vi "Limit Testing Frequency.vi"(6 "limit test config":T2={"pass region"=0, "include UL"=TRUE, "include LL"=TRUE} {"pass region" items=["inside limits", "outside limits"]}, 8 "error in (no error)":errorcluster, 9 "lower limit":cluster{"x0":dbl, "dx":dbl, "Y":dbl[]}={"x0"=0.0, "dx"=1.0, "Y"=[]} {"Y" format="%.2p"; "dx" format="%.2p"; "x0" format="%.2p"}, 10 "upper limit":cluster{"x0":dbl, "dx":dbl, "Y":dbl[]}={"x0"=0.0, "dx"=1.0, "Y"=[]} {"Y" format="%.2p"; "dx" format="%.2p"; "x0" format="%.2p"}, 11 "signal in":cluster{"f0":dbl, "df":dbl, "spectrum":dbl[]}={"f0"=0.0, "df"=1.0, "spectrum"=[]} {"spectrum" format="%.2p"; "df" format="%0.2p"; "f0" format="%0.2p"}) -> (0 "error out":errorcluster, 1 "output values":cluster{"x0":dbl, "dx":dbl, "Y":dbl[]}[](array[cluster]) {"Y" format="%.2p"; "dx" format="%.2p"; "x0" format="%.2p"}, 2 "test results":bool[](array[boolean]), 3 "test passed?":bool, 4 "clearance":T1 {"min clearance" format="%.2p"; "clearance LL" format="%.2p"; "clearance UL" format="%.2p"}, 5 "failures":cluster{"x values":dbl[], "y values":dbl[]} {"y values" format="%.2p"; "x values" format="%.2p"})   [LabVIEW 2020, in "NI_MAPro.lvlib"]
doc: "Performs limit testing on waveform or cluster input data. The VI compares <B>signal in</B> with <B>upper limit</B> and <B>lower limit</B> and ignores any limit input that is not wired. You can wire <B>output values</B> to a graph to view the limits, signal, and failures. Wire data to the <B>signal in</B> input to determine the polymorphic instance to use or manually select the instance."
uses:
  NI_MAPro.lvlib
  NI_MABase.lvlib
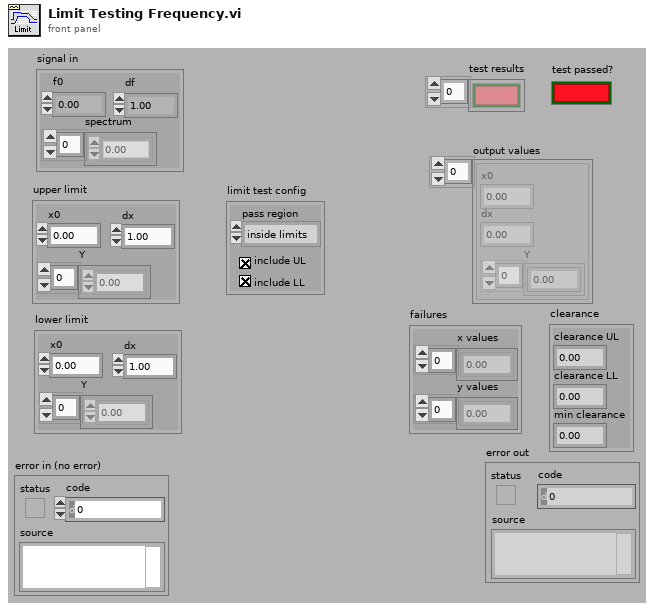
[diagram p1: front panel]
types:
  T1 = cluster{"clearance UL":dbl, "clearance LL":dbl, "min clearance":dbl}
  T2 = cluster{"pass region":i32, "include UL":bool, "include LL":bool}
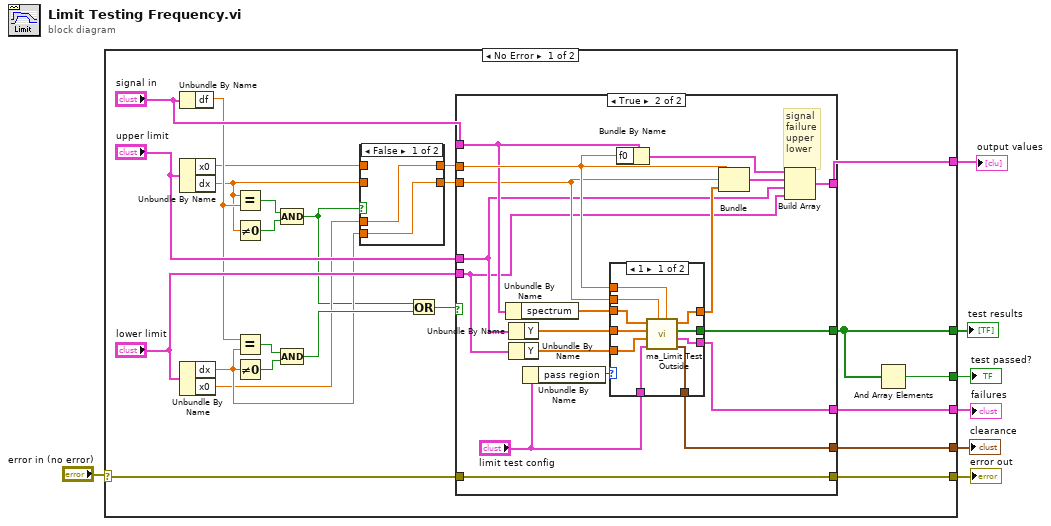
[diagram p0: block diagram]
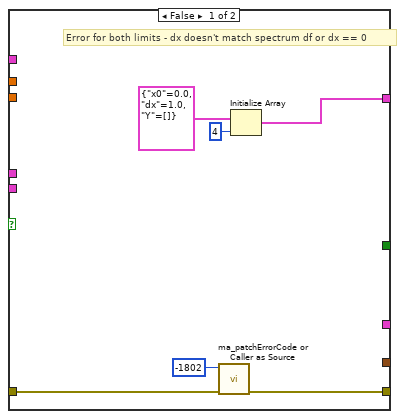
[diagram p3: hidden frame]
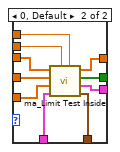
[diagram p4: hidden frame]
diagram:
  n1 = case shown="No Error" "error in (no error)" {
    selector: "error in (no error)" -> [w27 w80]
    tunnel: [w26 w80] -> w7
    tunnel: [w25 _] -> w6
    tunnel: [w20 _] -> w4
    tunnel: [w19 _] -> w3
    tunnel: [w18 _] -> w2
    tunnel: [w17 _] -> w1
    frame No Error {
      n2 = Unbundle By Name("signal in") -> ("df"=w21:dbl)
      n3 = Unbundle By Name("upper limit") -> ("x0"=w14:dbl, "dx"=w13:dbl)
      n4 = Unbundle By Name("lower limit") -> ("dx"=w12:dbl, "x0"=w11:dbl)
      n5 = Equal?(x=w13, y=w21) -> (x = y?=w30:bool)
      n6 = Not Equal To 0?(x=w13) -> (x != 0?=w29:bool)
      n7 = Equal?(x=w21, y=w12) -> (x = y?=w31:bool)
      n8 = Not Equal To 0?(x=w12) -> (x != 0?=w28:bool)
      n9 = Compound Arithmetic op=AND(w30, w29) -> (w8:bool)
      n10 = Compound Arithmetic op=AND(w31, w28) -> (w16:bool)
      n11 = case shown="False" w8 {
        tunnel: w14 -> [_ w35]
        tunnel: w13 -> [_ w34]
        tunnel: w11 -> [w33 _]
        tunnel: w12 -> [w32 _]
        tunnel: [w33 w35] -> w10
        tunnel: [w32 w34] -> w9
        frame False {
        }
        frame True {
        }
      }
      n12 = Or(x=w8, y=w16) -> (x .or. y?=w15:bool)
      n13 = case shown="True" w15 {
        tunnel: [_ w58] -> w20
        tunnel: "upper limit" -> [_ w46]
        tunnel: "lower limit" -> [_ w44]
        tunnel: "signal in" -> [_ w49]
        tunnel: w10 -> [_ w50]
        tunnel: w9 -> [_ w48]
        tunnel: w27 -> [w39 w42]
        tunnel: [w38 w42] -> w26
        tunnel: [w36 w59] -> w18
        tunnel: [_ w57] -> w25
        tunnel: [_ w56] -> w17
        frame False {
          # "Error for both limits - dx doesn't match spectrum df or dx == 0"
          n14 = call "ma_patchErrorCode or Caller as Source.vi"("error in (no error)"=w39, "error code"=-1802 ("Error Code")) -> ("error out"=w38:errorcluster)  [unwired: 2 in, 7 out]
          n15 = Initialize Array(cluster{"x0":dbl, "dx":dbl, "Y":dbl[]} {"x0"=0.0, "dx"=1.0, "Y"=[]} ("lower limit"), 4 ("dimension size")) -> (w36:cluster{"x0":dbl, "dx":dbl, "Y":dbl[]}[])
        }
        frame True {
          # "signal\nfailure\nupper\nlower"
          n16 = Unbundle By Name(w49) -> ("spectrum"=w47:dbl[])
          n17 = Unbundle By Name(w46) -> ("Y"=w45:dbl[])
          n18 = Unbundle By Name(w44) -> ("Y"=w43:dbl[])
          n19 = Unbundle By Name("limit test config") -> ("pass region"=w54:i32)
          n20 = case shown="1" w54 {
            tunnel: [w69 w73] -> w58
            tunnel: w45 -> [w68 w79]
            tunnel: w43 -> [w67 w78]
            tunnel: [w66 w77] -> w53
            tunnel: [w65 w76] -> w57
            tunnel: [w64 w75] -> w56
            tunnel: "limit test config" -> [w63 w74]
            tunnel: w50 -> [w62 w72]
            tunnel: w48 -> [w61 w71]
            tunnel: w47 -> [w60 w70]
            frame 1 {
              n21 = call "ma_Limit Test Outside.vi"("x0"=w62, "dx"=w61, "limit test config"=w63, "lower"=w67, "upper"=w68, "signal"=w60) -> ("clearance"=w64:T1, "failures"=w65:cluster{"x values":dbl[], "y values":dbl[]}, "test results"=w69:bool[], "Y"=w66:dbl[])  [unwired: 2 out]
            }
            frame 0, Default {
              n22 = call "ma_Limit Test Inside.vi"("x0"=w72, "dx"=w71, "limit test config"=w74, "lower"=w78, "upper"=w79, "signal"=w70) -> ("clearance"=w75:T1, "failures"=w76:cluster{"x values":dbl[], "y values":dbl[]}, "test results"=w73:bool[], "Y"=w77:dbl[])  [unwired: 2 out]
            }
          }
          n23 = Bundle By Name(cluster=w49, "f0"=w50) -> (w51:cluster{"f0":dbl, "df":dbl, "spectrum":dbl[]})
          n24 = Bundle("x0"=w50, "dx"=w48, "Y"=w53) -> (w52:cluster{"x0":dbl, "dx":dbl, "Y":dbl[]})  [unwired: 1 out]
          n25 = Build Array(w51, w52, w46, w44) -> (w59:cluster{"x0":dbl, "dx":dbl, "Y":dbl[]}[])
        }
      }
      n26 = And Array Elements(Boolean array=w20) -> (logical AND=w19:bool)
    }
    frame Error {
    }
  }
  "error out" <- w7
  "failures" <- w6
  "test passed?" <- w3
  "test results" <- w4
  "output values" <- w2
  "clearance" <- w1
